vi "tcs_getSample_kernelFK5Target.vi"(8 "error in (no error)":errorcluster, 11 "kernel_FK5Target_Ctl":T1) -> (0 "error out":errorcluster, 2 "function return":i32, 3 "kernel_FK5Target_Ctl out":T1)   [LabVIEW 2016, in "SALLV_tcs.lvlib"]
doc: "int tcs_shm_getSample_kernel_FK5TargetLV(tcs_kernel_FK5TargetLV *kernel_FK5Target_Ctl );"
uses:
  SALLV_tcs.lvlib
  DataTypes/kernel_FK5Target.ctl
  SALLV_tcs.so
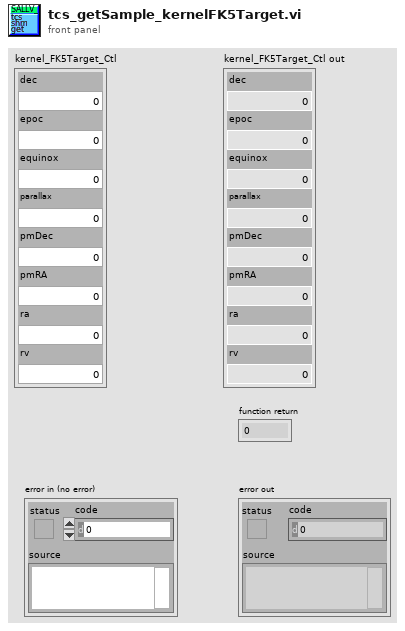
[diagram p1: front panel]
types:
  T1 = typedef "SALLV_tcs.lvlib/kernel_FK5Target.ctl" = cluster{"dec":sgl, "epoc":sgl, "equinox":sgl, "parallax":sgl, "pmDec":sgl, "pmRA":sgl, "ra":sgl, "rv":sgl}
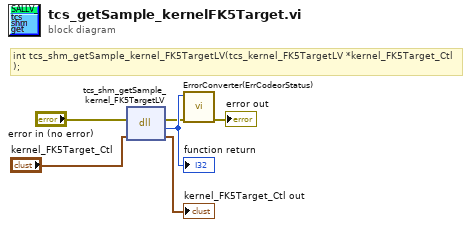
[diagram p0: block diagram]
diagram:
  # "int tcs_shm_getSample_kernel_FK5TargetLV(tcs_kernel_FK5TargetLV *kernel_FK5Target_Ctl );"
  n1 = dll-call lib="home/andres/Desktop/SALLV_tcs/SALLV_tcs.*" fn="tcs_shm_getSample_kernel_FK5TargetLV"(error in="error in (no error)", "kernel_FK5Target_Ctl"="kernel_FK5Target_Ctl") -> (error out=w2:errorcluster, w6:i32, "kernel_FK5Target_Ctl"=→"kernel_FK5Target_Ctl out":T1)  [unwired: 2 in, 1 out]
  "function return" <- w6
  n2 = call "ErrorConverter(ErrCodeorStatus).vi"("error in (no error)"=w2, "error code"=w6) -> ("error out"=→"error out":errorcluster)  [unwired: 9 in]
